vi "BRig_dataExp_Audio_amp_1B.vi"() -> (2 "output_Audio_amp__1B":i32)   [LabVIEW 2014]
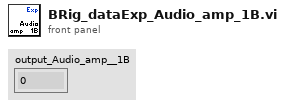
[diagram p1: front panel]
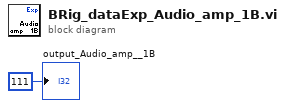
[diagram p0: block diagram]
diagram:
  "output_Audio_amp__1B" <- 111 ("output_iBlock")
